vi "Get subPanel Refnum.vi"(8 "error in (no error)":errorcluster, 11 "Panel Control_Ref in":refnum<class "Panel Controller.lvclass">) -> (0 "error out":errorcluster, 2 "Sub Panel Ref":refnum<vi>, 3 "Panel Control_Ref out":refnum<class "Panel Controller.lvclass">)   [LabVIEW 2015, in "Panel Controller.lvclass"]
uses:
  Panel Controller.lvclass
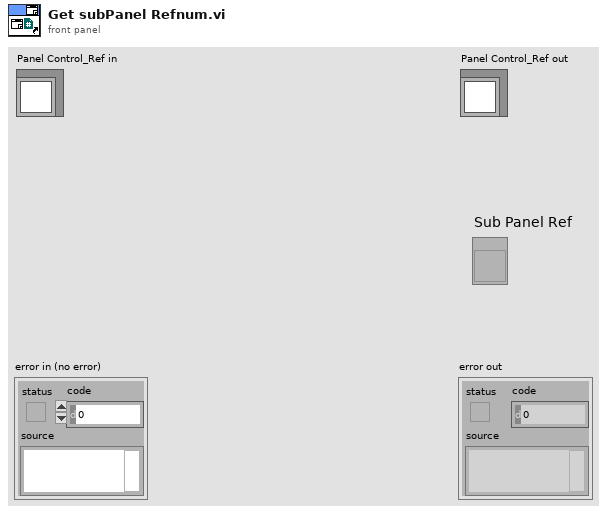
[diagram p1: front panel]
types:
  T1 = typedef "Panel Controller.lvclass/ObjectAttributes.ctl" = cluster{"Sub Panel Ref":refnum<vi>, "Panel_Q":refnum<queue>, "VI Running Refnum":refnum<vi>, "Brower Controller_Q":refnum<class "Message Enqueuer.lvclass">, "GUI Control Builder Director.lvclass":refnum<class "GUI Control Builder Director.lvclass">, "Panel GUI Manager.lvclass":refnum<class "Panel GUI Manager.lvclass">}
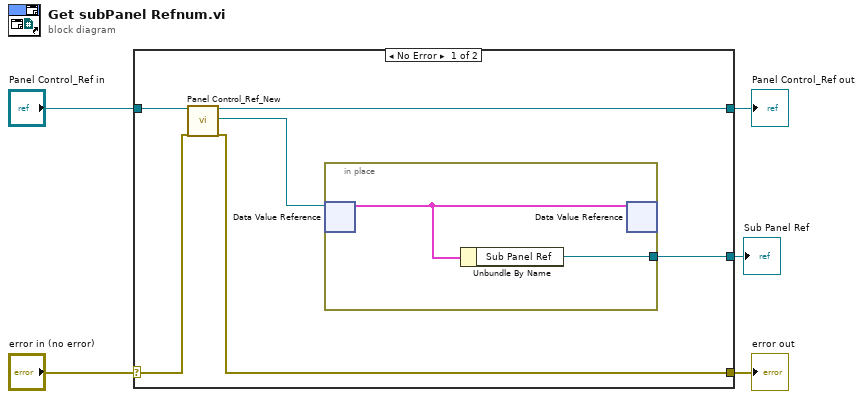
[diagram p0: block diagram]
diagram:
  n1 = case shown="No Error" "error in (no error)" {
    selector: "error in (no error)" -> [w8 w15]
    tunnel: [w7 w15] -> w4
    tunnel: [w9 w14] -> w2
    tunnel: "Panel Control_Ref in" -> [w10 w14]
    tunnel: [w6 _] -> w1
    frame No Error {
      n2 = call "Panel Control_Ref_New.vi"("reference in"=w10, "error in (no error)"=w8) -> ("reference out"=w9:refnum<class "Panel Controller.lvclass">, "DVRRefOut"=w11:refnum<data-value>, "error out"=w7:errorcluster)  [unwired: 14 in, 1 out]
      n3 = in-place {
        in-place-border: [w12] -> w6
        n4 = in-place-dvr #1(w11) -> (w13:T1)  [unwired: 1 out]
        n5 = Unbundle By Name(w13) -> ("Sub Panel Ref"=w12:refnum<vi>)
        n6 = in-place-dvr #1(w13) -> ()  [unwired: 2 out]
      }
    }
    frame Error {
    }
  }
  "error out" <- w4
  "Panel Control_Ref out" <- w2
  "Sub Panel Ref" <- w1
